vi "WriteAttributeTest.vi"(3 "device name":string="tango/tangotest/1") -> ()   [LabVIEW 2009]
uses:
  tango_lv8/tango_vi.llb/WriteShortScalarAttribute.vi
  tango_lv8/tango_vi.llb/WriteLongScalarAttribute.vi
  tango_lv8/tango_vi.llb/WriteDoubleScalarAttribute.vi
  tango_lv8/tango_vi.llb/WriteStringScalarAttribute.vi
panel:
  out "success":bool
  out "success":bool
  out "success":bool
  out "success":bool
  in  "value":dbl=123.456
  in  "attribute name":string="double_scalar"
  in  "value":i32=32768
  in  "attribute name":string="long_scalar"
  in  "value":i16=256
  in  "attribute name":string="short_scalar"
  in  "value":string="This is the write value..."
  in  "attribute name":string="string_scalar"
  # "TANGO  Binding for LabVIEW - WriteAttribute example"
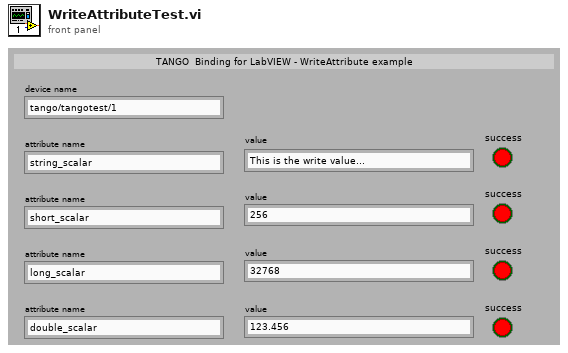
[diagram p1: front panel]
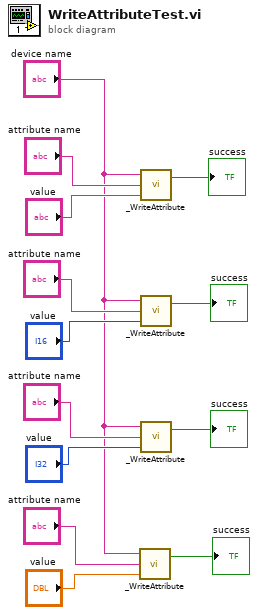
[diagram p0: block diagram]
diagram:
  n1 = call-poly "_WriteAttribute.vi"("value"="value", "attribute name"="attribute name", "device name"="device name") -> ("success"=→"success":bool)  [unwired: 1 out]
  n2 = call-poly "_WriteAttribute.vi"("value"="value", "attribute name"="attribute name", "device name"="device name") -> ("success"=→"success":bool)  [unwired: 1 out]
  n3 = call-poly "_WriteAttribute.vi"("value"="value", "attribute name"="attribute name", "device name"="device name") -> ("success"=→"success":bool)  [unwired: 1 out]
  n4 = call-poly "_WriteAttribute.vi"("value"="value", "attribute name"="attribute name", "device name"="device name") -> ("success"=→"success":bool)  [unwired: 1 out]
